vi "GetWindowSafeArea.vi"(8 "No Error":errorcluster, 11 "Window [SDL_Window *]":i64 format="%.0x") -> (0 "Error Out":errorcluster, 3 "Rect":T1)   [LabVIEW 2024, in "SDL3.lvlib" / "Video.lvlib"]
doc: "<B>Summary</B>\nGet the safe area for this window.\n\n<B>Remarks</B>\nSome devices have portions of the screen which are partially obscured or not interactive, possibly due to on-screen controls, curved edges, camera notches, TV overscan, etc. This function provides the area of the window which is safe to have interactable content. You should continue rendering into the rest of the window, but it should not contain visually important or interactible content."
uses:
  Video.lvlib
  Rect/Rect--cluster.ctl
  Rect/Rect.lvlib
  Lib/SDL3-32.dll
  Error/Error.lvlib
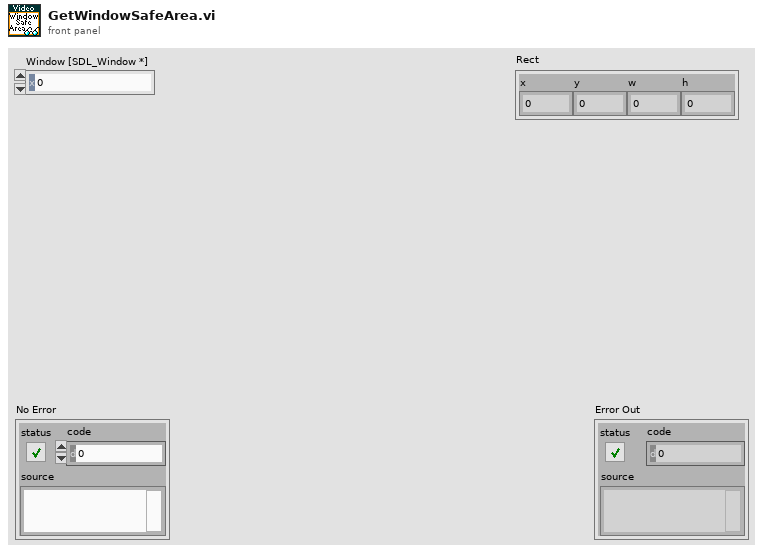
[diagram p1: front panel]
types:
  T1 = typedef "SDL3.lvlib/Rect.lvlib/Rect--cluster.ctl" = cluster{"x":i32, "y":i32, "w":i32, "h":i32}
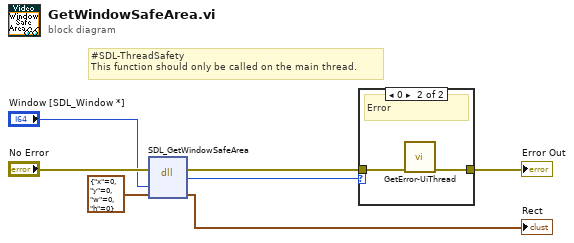
[diagram p0: block diagram]
diagram:
  # "#SDL-ThreadSafety\nThis function should only be called on the main thread."
  n1 = dll-call lib="C:/Users/Thomas/Documents/Projects/LV-SDL3/Lib/SDL3-*.*" fn="SDL_GetWindowSafeArea"(error in="No Error", "window"="Window [SDL_Window *]", "rect"=T1 {"x"=0, "y"=0, "w"=0, "h"=0} ("Rect")) -> (error out=w5:errorcluster, "return type"=w4:i32, "rect"=→"Rect":T1)  [unwired: 3 in, 1 out]
  n2 = case shown="0" w4 {
    tunnel: w5 -> [w8 w10]
    tunnel: [w8 w9] -> w3
    frame Default {
      # "Ok"
    }
    frame 0 {
      # "Error"
      n3 = call "GetError-UiThread.vi"("No Error"=w10) -> ("error out"=w9:errorcluster)  [unwired: 10 in]
    }
  }
  "Error Out" <- w3
